vi "ma_SML ND Zoom FFT (complex input).vi"(4 "error in (no error)":errorcluster, 5 "zoom settings":T2={"zoom settings"={"center frequency"=-inf, "zoom"=1, "trim"=1.0}, "FFT settings"={"window"=1, "FFT size"=-1}} {"FFT settings"."window" items=["Rectangle"=0, "Hanning"=1, "Hamming"=2, "Blackman-Harris"=3, "Exact Blackman"=4, "Blackman"=5, "Flat Top"=6, "4 Term B-Harris "=7, "7 Term B-Harris"=8, "Low Sidelobe"=9, "Blackman Nuttall"=11, "Triangle"=30, "Bartlett-Hanning"=31, "Bohman"=32, "Parzen"=33, "Welch"=34, "Kaiser"=60, "Dolph-Chebyshev"=61, "Gaussian"=62]; "zoom settings"."trim" min=1.0 format="%.2f"; "zoom settings"."center frequency" format="%.2f"; "zoom settings"."zoom" min=1}, 6 "fs":dbl=1024.0 format="%.2f", 7 "x":cdb[](array[numeric]) format="%.2f") -> (0 "error out":errorcluster, 2 "spectral info":T1 {"window" items=["Rectangle"=0, "Hanning"=1, "Hamming"=2, "Blackman-Harris"=3, "Exact Blackman"=4, "Blackman"=5, "Flat Top"=6, "4 Term B-Harris "=7, "7 Term B-Harris"=8, "Low Sidelobe"=9, "Blackman Nuttall"=11, "Triangle"=30, "Bartlett-Hanning"=31, "Bohman"=32, "Parzen"=33, "Welch"=34, "Kaiser"=60, "Dolph-Chebyshev"=61, "Gaussian"=62]}, 3 "FFT spectrum [Vrms]":T3 {"spectrum" format="%.2f"; "df" format="%.2f"; "f0" format="%.2f"})   [LabVIEW 2020, in "NI_MAPro.lvlib"]
uses:
  NI_MAPro.lvlib
  ma_sml_Spectrum Cluster (complex).ctl
  ma_sml_ND Zoom FFT Settings.ctl
  ma_sml_Spectral Info.ctl
  NI_AALPro.lvlib
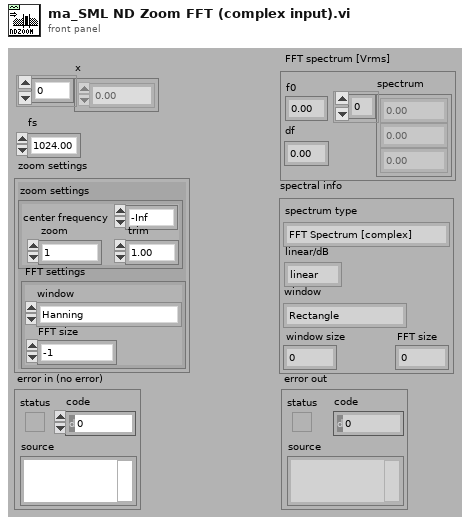
[diagram p1: front panel]
types:
  T1 = typedef "NI_MAPro.lvlib/ma_sml_Spectral Info.ctl" = cluster{"spectrum type":enum16{"FFT Spectrum [complex]", "Amplitude [Magnitude]", "Power [Magnitude^2]", "Cross Spectrum [complex]", "Frequency Response [Complex]"}, "linear/dB":enum16{"linear", "dB"}, "window":u16, "window size":i32, "FFT size":i32}
  T2 = typedef "NI_MAPro.lvlib/ma_sml_ND Zoom FFT Settings.ctl" = cluster{"zoom settings":cluster{"center frequency":dbl, "zoom":i32, "trim":dbl}, "FFT settings":cluster{"window":u16, "FFT size":i32}}
  T3 = typedef "NI_MAPro.lvlib/ma_sml_Spectrum Cluster (complex).ctl" = cluster{"f0":dbl, "df":dbl, "spectrum":cdb[]}
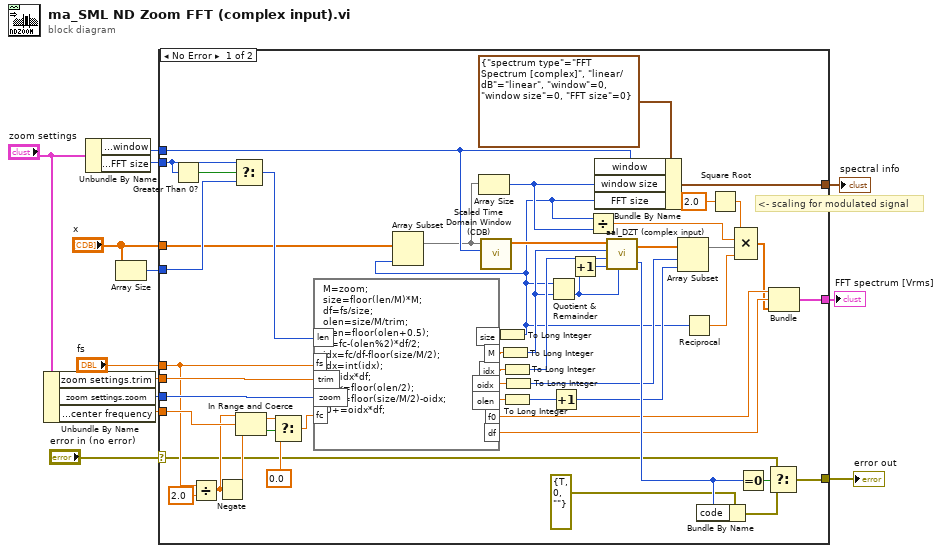
[diagram p0: block diagram]
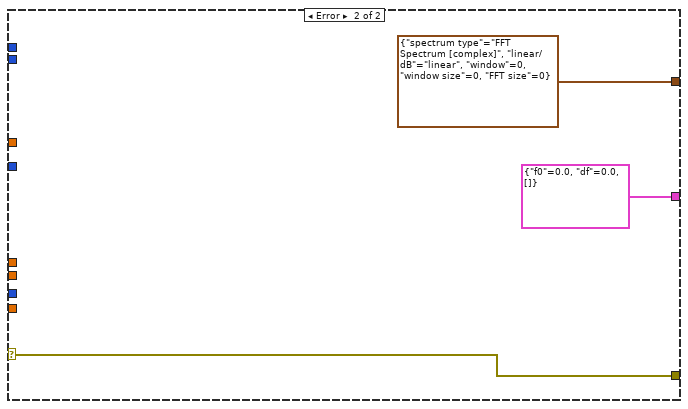
[diagram p2: hidden frame]
diagram:
  # "<- scaling for modulated signal"
  n1 = Unbundle By Name("zoom settings") -> ("zoom settings.trim"=w2:dbl, "zoom settings.zoom"=w4:i32, "zoom settings.center frequency"=w6:dbl)
  n2 = Unbundle By Name("zoom settings") -> ("FFT settings.window"=w3:u16, "FFT settings.FFT size"=w7:i32)
  n3 = Array Size(array="x") -> (size(s)=w5:i32)
  n4 = case shown="No Error" "error in (no error)" {
    selector: "error in (no error)" -> [w15 w66]
    tunnel: "x" -> [w18 _]
    tunnel: "fs" -> [w16 _]
    tunnel: [w61 cluster{"f0":dbl, "df":dbl, cdb[]} {"f0"=0.0, "df"=0.0, []}] -> w11
    tunnel: [w56 w66] -> w12
    tunnel: w3 -> [w48 _]
    tunnel: [w52 T1 {"spectrum type"=enum."FFT Spectrum [complex]", "linear/dB"=enum."linear", "window"=0, "window size"=0, "FFT size"=0} ("spectral info")] -> w10
    tunnel: w6 -> [w44 _]
    tunnel: w4 -> [w21 _]
    tunnel: w7 -> [w46 _]
    tunnel: w5 -> [w25 _]
    tunnel: w2 -> [w20 _]
    frame No Error {
      n5 = Greater Than 0?(x=w46) -> (x > 0?=w47:bool)
      n6 = Divide(x=w16, y=2.0) -> (x/y=w42:dbl)
      n7 = Negate(x=w42) -> (-x=w41:dbl)
      n8 = Select(t=w46, s=w47, f=w25) -> (s? t:f=w45:i32)
      n9 = In Range and Coerce(upper limit=w42, x=w44, lower limit=w41) -> (coerced(x)=w39:dbl, In Range?=w40:bool)
      n10 = Select(t=w39, s=w40, f=0.0) -> (s? t:f=w37:dbl)
      n11 = formula code="M=zoom;\nsize=floor(len/M)*M;\ndf=fs/size;\nolen=size/M/trim;\nolen=floor(olen+0.5);\nfc=fc-(olen%2)*df/2;\nidx=fc/df-floor(size/M/2);\nidx=int(idx);\nf0=idx*df;\noidx=floor(olen/2);\noidx=floor(size/M/2)-oidx;\nf0+=oidx*df;"("fs"=w16, "fc"=w37, "zoom"=w21, "len"=w45, "trim"=w20) -> ("f0"=w55:dbl, "df"=w54:dbl, "idx"=w62:dbl, "size"=w64:dbl, "M"=w63:dbl, "oidx"=w32:dbl, "olen"=w31:dbl)
      n12 = To Long Integer(number=w64) -> (32bit integer=w17:i32)
      n13 = Array Subset(array=w18, length=w17) -> (w19:cdb[])  [unwired: 1 in]
      n14 = Array Size(array=w19) -> (size(s)=w27:i32)
      n15 = call "Scaled Time Domain Window (CDB).vi"("window"=w48, "X"=w19) -> ("Windowed X"=w51:cdb[])  [unwired: 7 in, 2 out]
      n16 = To Long Integer(number=w63) -> (32bit integer=w49:i32)
      n17 = To Long Integer(number=w62) -> (32bit integer=w50:i32)
      n18 = To Long Integer(number=w31) -> (32bit integer=w29:i32)
      n19 = To Long Integer(number=w32) -> (32bit integer=w30:i32)
      n20 = Quotient & Remainder(x=w17, y=w49) -> (floor(x/y)=w22:i32)  [unwired: 1 out]
      n21 = Increment(x=w29) -> (x+1=w23:i32)
      n22 = Increment(x=w22) -> (x+1=w24:i32)
      n23 = Divide(x=w17, y=w27) -> (x/y=w26:dbl)
      n24 = Bundle By Name(cluster=T1 {"spectrum type"=enum."FFT Spectrum [complex]", "linear/dB"=enum."linear", "window"=0, "window size"=0, "FFT size"=0} ("spectral info"), "window"=w48, "window size"=w27, "FFT size"=w17) -> (w52:T1)
      n25 = call "aal_DZT (complex input).vi"("x"=w51, "M"=w49, "index"=w50, "out_len"=w24, "fft_len"=w22) -> ("Y"=w34:cdb[], "error"=w60:i32)
      n26 = Array Subset(array=w34, index=w30, length=w23) -> (w33:cdb[])
      n27 = Reciprocal(x=w17) -> (1/x=w36:dbl)
      n28 = Bundle By Name(cluster=errorcluster {"status"=TRUE, "code"=0, "source"=""} ("error in (no error)"), "code"=w60) -> (w58:errorcluster)
      n29 = Square Root(x=2.0 ("y")) -> (sqrt(x)=w28:dbl)
      n30 = Compound Arithmetic op=MULTIPLY(w28, w26, w33, w36) -> (w53:cdb[])
      n31 = Equal To 0?(x=w60) -> (x = 0?=w57:bool)
      n32 = Select(t=w15, s=w57, f=w58) -> (s? t:f=w56:errorcluster)
      n33 = Bundle("f0"=w55, "df"=w54, w53) -> (w61:cluster{"f0":dbl, "df":dbl, cdb[]})  [unwired: 1 out]
    }
    frame Error {
    }
  }
  "FFT spectrum [Vrms]" <- w11
  "error out" <- w12
  "spectral info" <- w10
